vi "amc_Send Message to Local Process.vi"(7 "Priority Message (F)":bool, 8 "error in (no error)":errorcluster, 10 "Message":T1, 11 "Process Name":string) -> (0 "error out":errorcluster)   [LabVIEW 2017]
uses:
  TypeDefs/amc_Message.ctl
  Tools/Keyed Array/Tools_KeyedArray KeyedArray.ctl
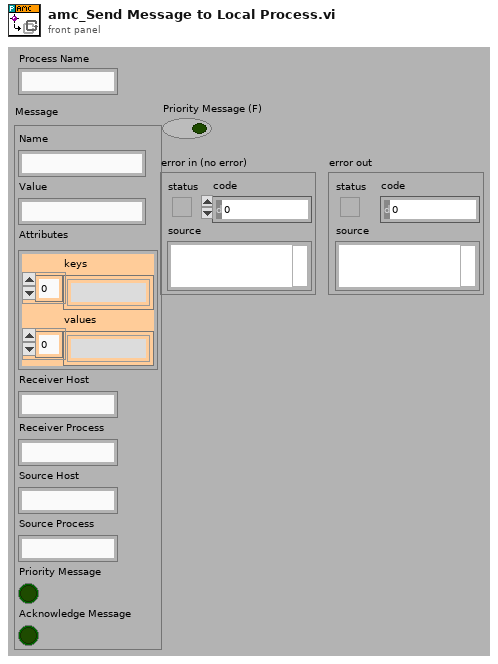
[diagram p1: front panel]
types:
  T1 = typedef "amc_Message.ctl" = cluster{"Name":string, "Value":string, "Attributes":T2, "Receiver Host":string, "Receiver Process":string, "Source Host":string, "Source Process":string, "Priority Message":bool, "Acknowledge Message":bool}
  T2 = typedef "Tools_KeyedArray KeyedArray.ctl" = cluster{"keys":string[], "values":string[]}
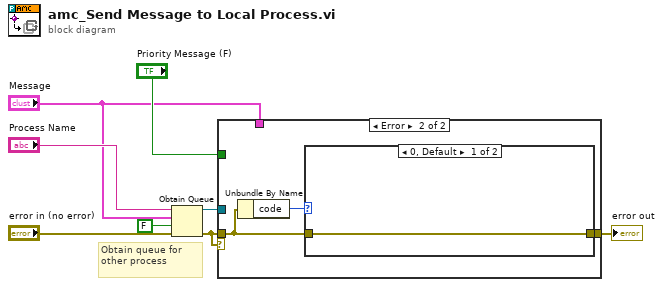
[diagram p0: block diagram]
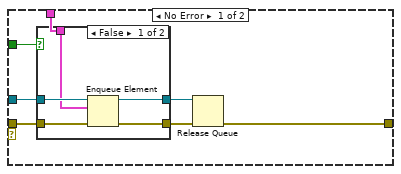
[diagram p2: hidden frame]
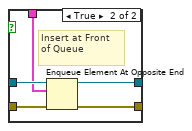
[diagram p3: hidden frame]
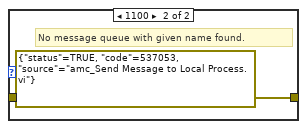
[diagram p4: hidden frame]
diagram:
  # "Obtain queue for\nother process"
  n1 = Obtain Queue(name (unnamed)="Process Name", element data type="Message", create if not found? (T)=FALSE, error in (no error)="error in (no error)") -> (queue out=w8:refnum<queue>, error out=w1:errorcluster)  [unwired: 1 in, 1 out]
  n2 = case shown="Error" w1 {
    tunnel: w1 -> [w15 w27]
    tunnel: w8 -> [w14 _]
    tunnel: [w12 w26] -> w6
    tunnel: "Priority Message (F)" -> [w10 _]
    tunnel: "Message" -> [w9 _]
    frame No Error {
      n3 = case shown="False" w10 {
        tunnel: w14 -> [w20 w24]
        tunnel: w15 -> [w19 w25]
        tunnel: [w17 w23] -> w11
        tunnel: w9 -> [w18 w22]
        tunnel: [w16 w21] -> w13
        frame False {
          n4 = Enqueue Element(queue=w20, element=w18, error in (no error)=w19) -> (queue out=w16:refnum<queue>, error out=w17:errorcluster)  [unwired: 2 out]
        }
        frame True {
          # "Insert at Front\nof Queue"
          n5 = Enqueue Element At Opposite End(queue=w24, element=w22, error in (no error)=w25) -> (queue out=w21:refnum<queue>, error out=w23:errorcluster)  [unwired: 2 out]
        }
      }
      n6 = Release Queue(queue=w13, error in (no error)=w11) -> (error out=w12:errorcluster)  [unwired: 3 out]
    }
    frame Error {
      n7 = Unbundle By Name(w27) -> ("code"=w28:i32)
      n8 = case shown="0, Default" w28 {
        tunnel: [w29 errorcluster {"status"=TRUE, "code"=537053, "source"="amc_Send Message to Local Process.vi"} ("error out")] -> w26
        tunnel: w27 -> [w29 _]
        frame 0, Default {
        }
        frame 1100 {
          # "No message queue with given name found."
        }
      }
    }
  }
  "error out" <- w6
